vi "AlphaBetaToABC_PowerInvariant_src.vi"(0 "alpha":sgl format="%#_32g", 5 "beta":sgl format="%#_32g") -> (4 "A":sgl format="%#_32g", 6 "B":sgl, 8 "C":sgl)   [LabVIEW 2015]
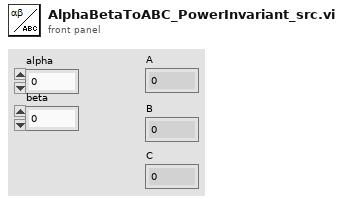
[diagram p1: front panel]
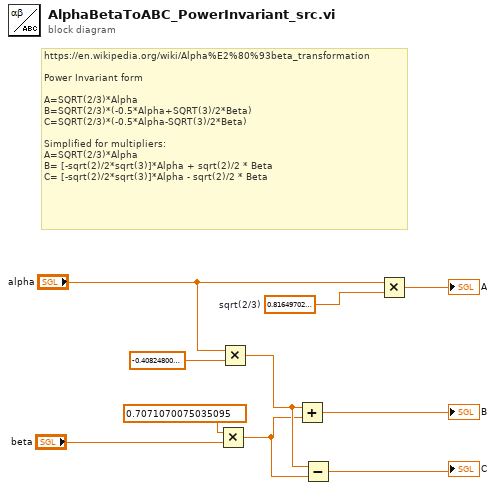
[diagram p0: block diagram]
diagram:
  w4 = sgl 0.816497  # sqrt(2/3)
  # "https://en.wikipedia.org/wiki/Alpha%E2%80%93beta_transformation\n\nPower Invariant form\n\nA=SQRT(2/3)*Alpha\nB=SQRT(2/3)*(-0.5*Alpha+SQRT(3)/2*Beta)\nC=SQRT(2/3)*(-0.5*Alpha-SQRT(3)/2*Beta)\n\nSimplified for multipliers:\nA=SQRT(2/3)*Alpha\nB= [-sqrt(2)/2*sqrt(3)]*Alpha + sqrt(2)/2 * Beta\nC= [-sqrt(2)/2*sqrt(3)]*Alpha - sqrt(2)/2 * Beta"
  n1 = Multiply(x=sgl 0.707107 ("beta"), y="beta") -> (x*y=w1:sgl)
  n2 = Multiply(x="alpha", y=sgl -0.408248) -> (x*y=w2:sgl)
  n3 = Add(x=w2, y=w1) -> (x+y=→"B":sgl)
  n4 = Subtract(x=w2, y=w1) -> (x-y=→"C":sgl)
  n5 = Multiply(x="alpha", y=w4) -> (x*y=→"A":sgl)
